vi "RemoveDuplicatElem.vi"(1 "Input Array":string[](array[string]), 2 "Remove Empty Strings?":bool) -> (0 "Discrete Array":string[](array[string]))   [LabVIEW 2015]
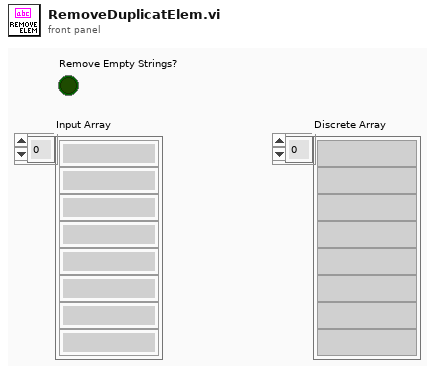
[diagram p1: front panel]
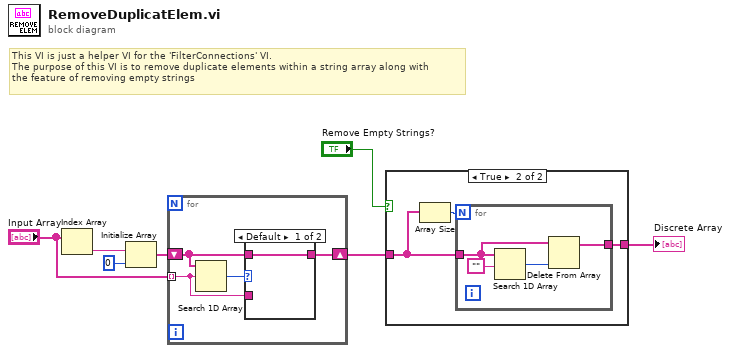
[diagram p0: block diagram]
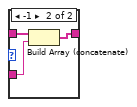
[diagram p3: hidden frame]
diagram:
  # "This VI is just a helper VI for the 'FilterConnections' VI.\nThe purpose of this VI is to remove duplicate elements within a string array along with\nthe feature of removing empty strings"
  n1 = Index Array(array="Input Array") -> (element=w4:string)  [unwired: 1 in]
  n2 = Initialize Array(w4, 0 ("dimension size")) -> (w6:string[])
  n3 = for {
    tunnel: "Input Array" -> [w10] mode=indexing
    shift-right: [w8] -> w2
    shift-left: w6 -> [w9]
    n4 = Search 1D Array(1D array=w9, element=w10) -> (index of element=w11:i32)  [unwired: 1 in]
    n5 = case shown="Default" w11 {
      tunnel: w10 -> [_ w14]
      tunnel: w9 -> [w12 w15]
      tunnel: [w12 w13] -> w8
      frame Default {
      }
      frame -1 {
        n6 = Build Array (concatenate)(w15, w14) -> (w13:string[])
      }
    }
  }
  n7 = case shown="True" "Remove Empty Strings?" {
    tunnel: [w16 w17] -> w1
    tunnel: w2 -> [w16 w18]
    frame False {
    }
    frame True {
      n8 = Array Size(array=w18) -> (size(s)=w19:i32)
      n9 = for {
        N: w19 -> [_]
        tunnel: w18 -> [w22]
        tunnel: [w20] -> w17
        n10 = Search 1D Array(1D array=w22, element="") -> (index of element=w21:i32)  [unwired: 1 in]
        n11 = Delete From Array(array=w22, index=w21) -> (array with subset deleted=w20:string[])  [unwired: 1 in, 1 out]
      }
    }
  }
  "Discrete Array" <- w1
